vi "LTC-20-Correction(B) v0.3.vi"(2 "Rat(dlogR/dlogT)":dbl=0.66 format="%.2f", 3 "Current Field":dbl=9.0 format="%.2f", 4 "Desired Temperature":dbl=305.0 format="%.2f") -> (0 "Correction Coef.":dbl format="%.2f", 1 "TempSetpoint":dbl=308.355 format="%.2f")   [LabVIEW 2024]
panel:
  out "?":cluster{dbl[], dbl[]} {"?" format="%.2f"; "?" format="%.2f"}
  in  "TempVals":dbl[][](array[numeric])=[[0.0, 4.239999771118164, 5.046999931335449, 5.98199987411499, 7.918000221252441, 10.376999855041504, 15.005000114440918, 20.309999465942383, 30.100000381469727], [0.0, 0.0, 0.0, 0.0, 0.0, 0.0, 0.0, 0.0, 0.0], [2.0, 0.0, -0.10499999672174454, -0.09700000286102295, -0.05700000002980232, -0.05700000002980232, -0.03400000184774399, -0.03500000014901161, -0.008999999612569809], [4.0, 0.0, -0.10400000214576721, -0.014000000432133675, 0.01899999938905239, -0.01600000075995922, -0.039000000804662704, -0.04500000178813934, -0.02199999988079071], [6.0, 0.0, 0.04600000008940697, 0.15600000321865082, 0.22100000083446503, 0.125, 0.014999999664723873, -0.04699999839067459, -0.029999999329447746], [8.0, 0.0, 0.375, 0.44600000977516174, 0.5059999823570251, 0.33799999952316284, 0.11400000005960464, -0.014999999664723873, -0.032999999821186066], [10.0, 0.0, 0.7990000247955322, 0.859000027179718, 0.8640000224113464, 0.6019999980926514, 0.24899999797344208, 0.03500000014901161, -0.03500000014901161], [12.0, 0.0, 1.24399995803833, 1.2970000505447388, 1.2389999628067017, 0.902999997138977, 0.3959999978542328, 0.09399999678134918, -0.03700000047683716], [14.0, 0.0, 1.5740000009536743, 1.6699999570846558, 1.6169999837875366, 1.1799999475479126, 0.5379999876022339, 0.1469999998807907, -0.039000000804662704], [16.0, 0.0, 1.8259999752044678, 1.9869999885559082, 1.9589999914169312, 1.4160000085830688, 0.6690000295639038, 0.1979999989271164, -0.050999999046325684], [18.0, 0.0, 1.9800000190734863, 2.236999988555908, 2.194999933242798, 1.621000051498413, 0.781000018119812, 0.23999999463558197, -0.06700000166893005], [20.0, 0.0, 1.9670000076293945, 2.2709999084472656, 2.2899999618530273, 1.7369999885559082, 0.8669999837875366, 0.267, -0.08799999952316284], [22.0, 0.0, 1.94, 2.3, 2.3, 1.78, 0.867, 0.267, -0.088], [24.0, 0.0, 1.94, 2.3, 2.3, 1.78, 0.867, 0.267, -0.088], [26.0, 0.0, 1.94, 2.3, 2.3, 1.78, 0.867, 0.267, -0.088], [28.0, 0.0, 1.94, 2.3, 2.3, 1.78, 0.867, 0.267, -0.088], [30.0, 0.0, 1.94, 2.3, 2.3, 1.78, 0.867, 0.267, -0.088]] format="%.5f"
  out "TempCorr":dbl[](array[numeric])=[1.0, 0.999, 0.997, 0.998, 1.008, 1.014, 1.015, 1.0195, 1.022, 1.024, 1.027, 1.03, 1.0335, 1.037, 1.04, 1.044, 1.048, 1.0525, 1.0567, 1.06, 1.064, 1.068, 1.07, 1.073, 1.078, 1.088] format="%.5f"
  out "Field":dbl[](array[numeric])=[0.0, 2.0, 4.0, 6.0, 8.0, 10.0, 11.0, 12.0, 13.0, 14.0, 15.0, 16.0, 17.0, 18.0, 19.0, 20.0, 21.0, 22.0, 23.0, 24.0, 25.0, 26.0, 27.0, 28.0, 29.0, 30.0] format="%.2f"
  out "TCArray":dbl[][](array[numeric])=[[0.0, 2.0, 4.0, 6.0, 8.0, 10.0, 11.0, 12.0, 13.0, 14.0, 15.0, 16.0, 17.0, 18.0, 19.0, 20.0, 21.0, 22.0, 23.0, 24.0, 25.0, 26.0, 27.0, 28.0, 29.0, 30.0], [0.0, -0.1, -0.3, -0.2, 0.8, 1.4, 1.5, 1.95, 2.2, 2.4, 2.7, 3.0, 3.35, 3.7, 4.0, 4.4, 4.8, 5.25, 5.67, 6.0, 6.4, 6.8, 7.0, 7.3, 7.8, 8.8]] format="%.4f"
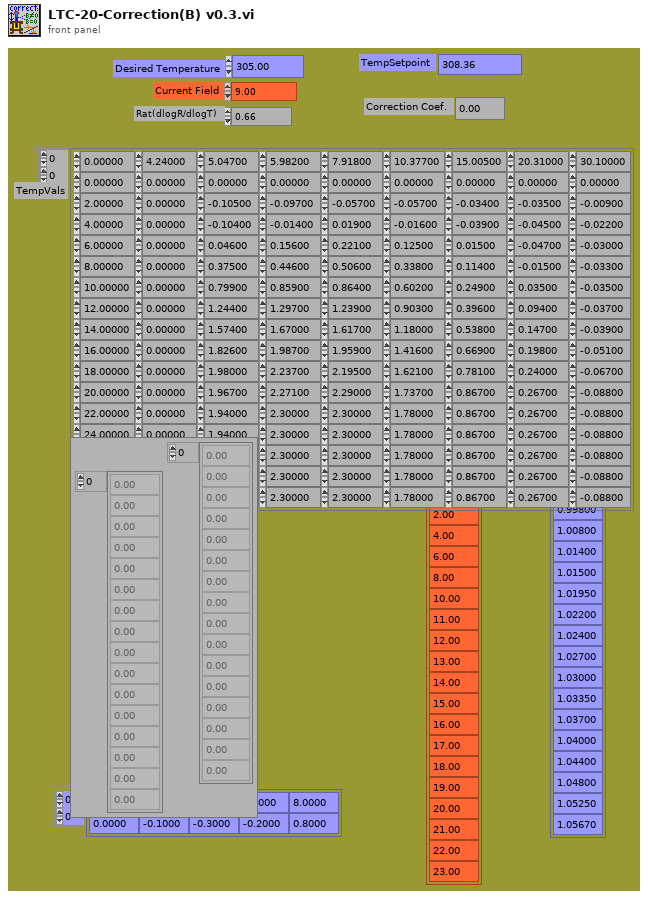
[diagram p1: front panel]
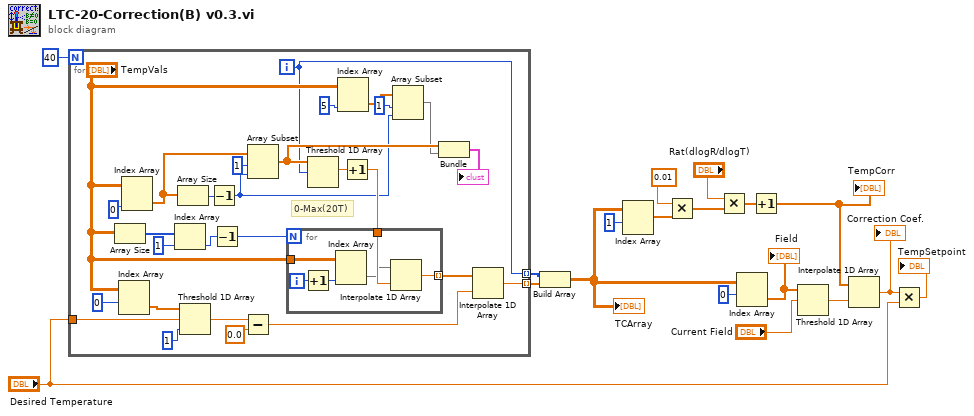
[diagram p0: block diagram]
diagram:
  n1 = for {
    N: 40 -> [_]
    tunnel: [w41] -> w17 mode=indexing
    tunnel: "Desired Temperature" -> [w39]
    tunnel: [w19] -> w16 mode=indexing
    i -> [w19]
    # "0-Max(20T)"
    n2 = Array Size(array="TempVals") -> (size(s)=w43:i32[])
    n3 = Index Array(array="TempVals", index (row)=0) -> (element=w30:dbl[])  [unwired: 1 in]
    n4 = Index Array(array="TempVals", index (col)=0) -> (element=w26:dbl[])  [unwired: 1 in]
    n5 = Index Array(array=w43, index=1) -> (element=w35:i32)
    n6 = Array Size(array=w26) -> (size(s)=w44:i32)
    n7 = Threshold 1D Array(1:1, 2:w39, 3:w30) -> (0:w32:dbl)
    n8 = Decrement(x=w44) -> (x-1=w21:i32)
    n9 = Decrement(x=w35) -> (x-1=w33:i32)
    n10 = Subtract(x=w32, y=0.0) -> (x-y=w31:dbl)
    n11 = Array Subset(array=w26, index=1, length=w21) -> (w28:dbl[])
    n12 = Threshold 1D Array(2:w19, 3:w28) -> (0:w40:dbl)  [unwired: 1 in]
    n13 = Index Array(array="TempVals", index (col)=5) -> (element=w24:dbl[])  [unwired: 1 in]
    n14 = Increment(x=w40) -> (x+1=w37:dbl)
    n15 = for {
      N: w33 -> [_]
      tunnel: w37 -> [w52]
      tunnel: [w51] -> w29 mode=indexing
      tunnel: "TempVals" -> [w50]
      i -> [w49]
      n16 = Increment(x=w49) -> (x+1=w48:i32)
      n17 = Index Array(array=w50, index (col)=w48) -> (element=w47:dbl[])  [unwired: 1 in]
      n18 = Interpolate 1D Array(1:w52, 2:w47) -> (0:w51:dbl)
    }
    n19 = Array Subset(array=w24, index=1, length=w21) -> (w22:dbl[])
    n20 = Bundle(w28, w22) -> (→"?":cluster{dbl[], dbl[]})  [unwired: 1 in]
    n21 = Interpolate 1D Array(1:w31, 2:w29) -> (0:w41:dbl)
  }
  n22 = Build Array(w16, w17) -> (w15:dbl[][])
  "TCArray" <- w15
  n23 = Index Array(array=w15, index (row)=1) -> (element=w6:dbl[])  [unwired: 1 in]
  n24 = Multiply(x=0.01, y=w6) -> (x*y=w3:dbl[])
  n25 = Multiply(x="Rat(dlogR/dlogT)", y=w3) -> (x*y=w5:dbl[])
  n26 = Index Array(array=w15, index (row)=0) -> (element=w10:dbl[])  [unwired: 1 in]
  "Field" <- w10
  n27 = Increment(x=w5) -> (x+1=w2:dbl[])
  "TempCorr" <- w2
  n28 = Threshold 1D Array(2:"Current Field", 3:w10) -> (0:w13:dbl)  [unwired: 1 in]
  n29 = Interpolate 1D Array(1:w13, 2:w2) -> (0:w1:dbl)
  "Correction Coef." <- w1
  n30 = Multiply(x=w1, y="Desired Temperature") -> (x*y=→"TempSetpoint":dbl)
